vi "PS90_Connect.vi"(1 "par5":i32, 2 "par2":i32=9600, 4 "par6":i32 min=0 max=1000, 5 "Interface":i32, 6 "par4":i32, 7 "Control unit ID":i32=1 min=1 max=20, 8 "error in (no error)":errorcluster, 9 "par3":i32, 10 "par1":i32=1, 11 "DLOwis.lvclass":refnum<class "DLOwis.lvclass">) -> (0 "error out":errorcluster, 3 "DLOwis.lvclass":refnum<class "DLOwis.lvclass">)   [LabVIEW 2019, in "DLOwis.lvclass"]
doc: "PS90_Connect.vi, created: 06.10.2006 alex; last change: 18.07.2016 alex;\n\n<B>FUNCTION:</B> \n\nOpen interface and connect to PS 90.\n*Serial interface (communication via USB or serial port)*\nThe application software can access this interface in the same way as \nit would access a standard serial port (COM). The parameters for Baudrate, \nParity, Databits and Stopbits are predefined (9600, no parity, 8 databits, 1 stopbit).\nThe software handshake character is CR.\n*Ethernet interface (communication via Com-Server)*\nAs Com-Server the OWIS software tool \"OWISerialServer.exe\" may be used\n(..\\OWISoft\\Application\\system). Alternatively, you can use other commercial\nproducts (hardware/software). The application software can access this interface\nvia Windows TCP socket: \nspecial communication for OWIS software (command + delay);\ncommon communication for other software/hardware (command).\nThe software handshake character is CR.\n*Ethernet interface (communication via Modbus/TCP Anybus-module)*\nThe application software can access this interface via Modbus/TCP socket (port=502).\n----------------------------------------------------------------------------------------\n<B>INPUT:</B>\n[I32] <B>Control unit ID:</B> control unit index 1-10. (Default=1, Range=1...20) \n11...20 - debug mode\n1...10 - standard mode\n[I32] <B>Interface:</B> define interface. (Default=0)\nUSB or serial port (=0)\n[I32] <B>par1:</B> define COM port. (Default=1 - COM1, Range=0...255) \n[I32] <B>par2:</B> define request mode for communication. (Default=9600) \n115200 - fast read (all bytes, fast check)\n19200 - fast read (all bytes, slow check)\n9600* - standard read (byte-by-byte)\n[I32] <B>par3:</B> define delay value (=20+x) for serial communication. \n(Default=20 ms) \n[I32] <B>par4:</B> system value. (Default=0) \n10 - without check\n0* - with check (firmware, terminal mode, clear error)\n[I32] <B>par5:</B> system value. (Default=0) \n10 - with port flush\n0* - without port flush\n[I32] <B>par6:</B> system value. (Default=0) \n5 - reconnect for every message\n0* - without reconnect\nEthernet interface + delay in ms (=20+x)\n[I32] <B>par1:</B> define ip address (block 1). (Default=0, Range=0...255) \n[I32] <B>par2:</B> define ip address (block 2). (Default=0, Range=0...255) \n[I32] <B>par3:</B> define ip address (block 3). (Default=0, Range=0...255) \n[I32] <B>par4:</B> define ip address (block 4). (Default=0, Range=0...255) \n[I32] <B>par5:</B> define port number. (Default=1200, Modbus/TCP=502) \n[I32] <B>par6:</B> system value or timeout value in ms for Modbus/TCP. \n(Default=0, Modbus/TCP=100) \nCom-Server\n5 - activate reconnect for every message (option 1)\n6 - activate common communication for other software/hardware (option 2)\n7 - activate both options (1 & 2)\n0* - deactivate both options (1 & 2)\n- without reconnect\n- special communication for OWIS software\n10...20 - without check\n0* - with check\nModbus/TCP\n5 - activate reconnect for every message (timeout=100 ms)\n0* - deactivate reconnect, timeout value\n[CLU] <B>error in</B>\n* - all other values.\n----------------------------------------------------------------------------------------\n<B>OUTPUT:</B>\n[CLU] <B>error out</B>\n0 - no error\n1 - function error (invalid parameters),\n3 - invalid serial port (port is not found),\n4 - access denied (port is busy),\n5 - no response from control unit (check cable, connection or reset control unit),\n8 - no connection to modbus/tcp,\n9 - no connection to tcp/ip socket.\n----------------------------------------------------------------------------------------\n<B>SUB-VIs:</B>\n----------------------------------------------------------------------------------------\n<B>EXT-Calls:</B>\nps90.dll (V2.00)\n----------------------------------------------------------------------------------------"
uses:
  DLOwis.lvclass
  C:/Dev/TRANCON/Classes/Delay Line/DelayLine.lvclass
  DelayLine.lvclass/DelayLine.ctl
  DelayLine.lvclass
panel:
  # "Interface:\n0 - serial                 1(+x) - ethernet (+ delay in ms)"
  # "COM port:\n0 - COM0\n1 - COM1\n..........\n255 - COM255"
  # "IP address:\nblock 1 (0...255)"
  # "Baudrate:\n9600\n19200\n38400\n57600\n115200"
  # "IP address:\nblock 2 (0...255)"
  # "IP address:\nblock 3 (0...255)"
  # "Delay:\nin ms"
  # "IP address:\nblock 4 (0...255)"
  # "Network port:\n1200 (Serial Server)\n 502 (Modbus/TCP)"
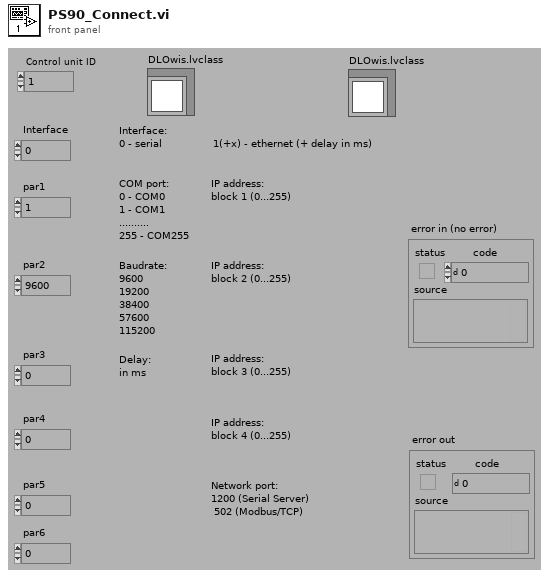
[diagram p1: front panel]
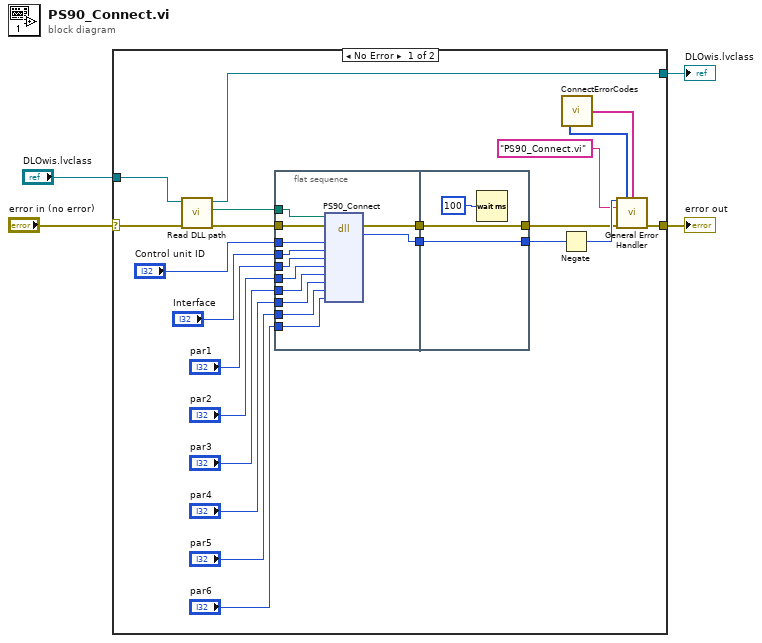
[diagram p0: block diagram]
diagram:
  n1 = case shown="No Error" "error in (no error)" {
    selector: "error in (no error)" -> [w8 w42]
    tunnel: [w19 w42] -> w4
    tunnel: "DLOwis.lvclass" -> [w10 w43]
    tunnel: [w9 w43] -> w2
    frame No Error {
      n2 = call "Read DLL path.vi"("error in (no error)"=w8, "DelayLine in"=w10) -> ("error out"=w12:errorcluster, "DLL path"=w7:path, "DelayLine out"=w9:refnum<class "DLOwis.lvclass">)  [unwired: 7 in]
      n3 = flat-sequence {
        tunnel: "par5" -> [w38]
        tunnel: "par4" -> [w37]
        tunnel: "par3" -> [w36]
        tunnel: "par2" -> [w35]
        tunnel: "par1" -> [w34]
        tunnel: "Interface" -> [w33]
        tunnel: "Control unit ID" -> [w32]
        tunnel: "par6" -> [w30]
        tunnel: w12 -> [w29]
        tunnel: w7 -> [w27]
        tunnel: [w31] -> w6
        tunnel: [w28] -> w5
        tunnel: [w40] -> w11
        tunnel: [w41] -> w18
        tunnel: w6 -> [w41]
        tunnel: w5 -> [w40]
        frame #0 {
          n4 = dll-call lib="C:/Dev/TRANCON/DLL/ps90.dll" fn="PS90_Connect"(path in=w27, error in=w29, "Index"=w32, "Interface"=w33, "par1"=w34, "par2"=w35, "par3"=w36, "par4"=w37, "par5"=w38, "par6"=w30) -> (error out=w28:errorcluster, "Rückgabetyp"=w31:i32)  [unwired: 9 in, 1 out]
        }
        frame #1 {
          n5 = Wait (ms)(milliseconds to wait=u32 100) -> ()  [unwired: 1 out]
        }
      }
      n6 = Negate(x=w18) -> (-x=w16:i32)
      n7 = call "ConnectErrorCodes.vi"() -> ("[user-defined descriptions]"=w13:string[], "[user-defined codes]"=w14:i32[])
      n8 = call <vilib>:"General Error Handler.vi"("[error code] (0)"=w16, "[user-defined codes]"=w14, "[user-defined descriptions]"=w13, "[error source] (\" \")"="PS90_Connect.vi", "error in (no error)"=w11) -> ("error out"=w19:errorcluster)  [unwired: 6 in, 4 out]
    }
    frame Error {
    }
  }
  "error out" <- w4
  "DLOwis.lvclass" <- w2
